vi "Configure Timebase (Basic).vi"(0 "VISA resource name":refnum<visa-resource-name>, 1 "Reference (1: Center)":i32(ring)=1 items=["Left", "Center", "Right"], 2 "Enable Vernier (F: Disable)":bool, 5 "Time Base Type (0: Main)":i32(ring) items=["Main", "Window", "XY", "Roll"], 7 "Scale (50 s/div)":dbl=50.0, 9 "Range (0.001 S)":dbl=0.001, 11 "error in (no error)":errorcluster, 12 "Position (0.0)":dbl, 13 "Enable REF BNC (F: Disable)":bool) -> (4 "VISA resource name out":refnum<visa-resource-name>, 15 "error out":errorcluster)   [LabVIEW 2016, in "Agilent 2000 3000 X-Series.lvlib"]
doc: "Configure the basic settings of time base."
uses:
  Agilent 2000 3000 X-Series.lvlib
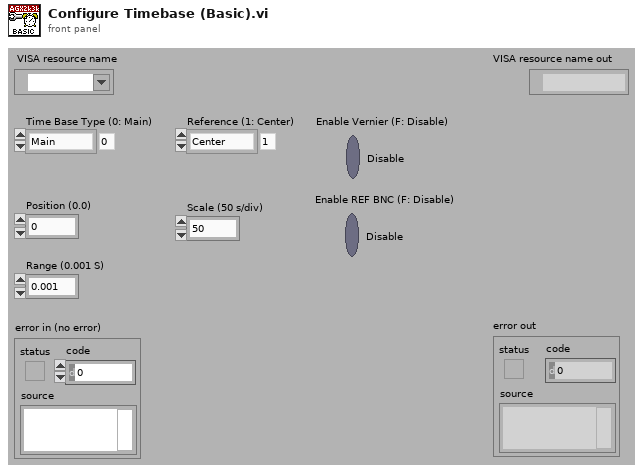
[diagram p1: front panel]
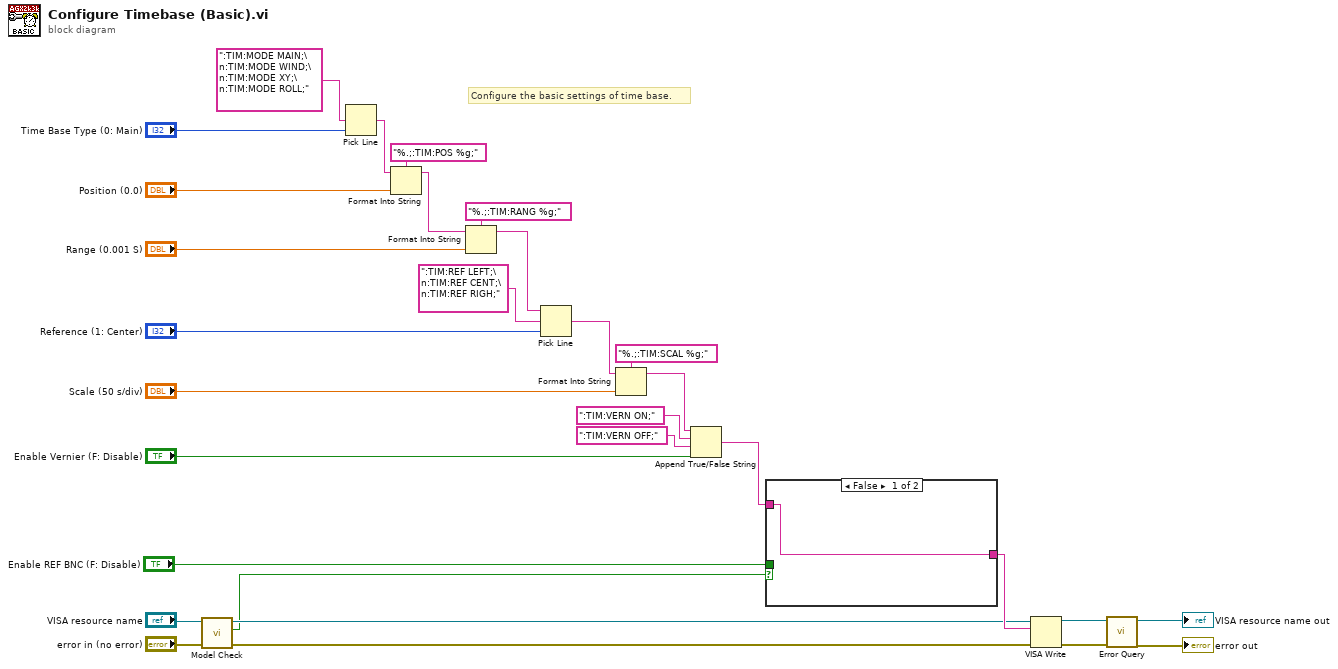
[diagram p0: block diagram]
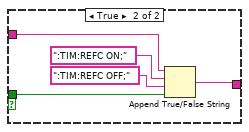
[diagram p2: hidden frame]
diagram:
  # "Configure the basic settings of time base."
  n1 = call "Model Check.vi"("error in (no error)"="error in (no error)", "VISA resource name"="VISA resource name") -> ("error out"=w2:errorcluster, "Not 2000 or 3000 Series"=w1:bool, "VISA resource name out"=w3:refnum<visa-resource-name>)  [unwired: 7 out]
  n2 = Pick Line(multi-line string=":TIM:MODE MAIN;\n:TIM:MODE WIND;\n:TIM:MODE XY;\n:TIM:MODE ROLL;", line index="Time Base Type (0: Main)") -> (output string=w28:string)  [unwired: 1 out]
  n3 = Format Into String(format string="%.;:TIM:POS %g;", initial string=w28, "Position (0.0)") -> (resulting string=w25:string)  [unwired: 1 in, 1 out]
  n4 = Format Into String(format string="%.;:TIM:RANG %g;", initial string=w25, "Range (0.001 S)") -> (resulting string=w20:string)  [unwired: 1 in, 1 out]
  n5 = Pick Line(string ("")=w20, multi-line string=":TIM:REF LEFT;\n:TIM:REF CENT;\n:TIM:REF RIGH;", line index="Reference (1: Center)") -> (output string=w19:string)
  n6 = Format Into String(format string="%.;:TIM:SCAL %g;", initial string=w19, "Scale (50 s/div)") -> (resulting string=w16:string)  [unwired: 1 in, 1 out]
  n7 = Append True/False String(1:"Enable Vernier (F: Disable)", 2:":TIM:VERN OFF;", 3:":TIM:VERN ON;", 4:w16) -> (0:w8:string)
  n8 = case shown="False" w1 {
    tunnel: w8 -> [w31 w34]
    tunnel: "Enable REF BNC (F: Disable)" -> [_ w33]
    tunnel: [w31 w32] -> w6
    frame False {
    }
    frame True {
      n9 = Append True/False String(1:w33, 2:":TIM:REFC OFF;", 3:":TIM:REFC ON;", 4:w34) -> (0:w32:string)
    }
  }
  n10 = VISA Write(VISA resource name=w3, write buffer=w6, error in (no error)=w2) -> (VISA resource name out=w12:refnum<visa-resource-name>, error out=w11:errorcluster)  [unwired: 1 out]
  n11 = call "Error Query.vi"("error in (no error)"=w11, "VISA resource name"=w12) -> ("error out"=→"error out":errorcluster, "VISA resource name out"=→"VISA resource name out":refnum<visa-resource-name>)  [unwired: 8 out]
